vi "Send Parameter To ParameterDevice.vi"(8 "error in (no error)":errorcluster, 10 "Value":dbl, 11 "ExperimentService in":refnum<class "ExperimentService.lvclass">) -> (0 "error out":errorcluster, 3 "ExperimentService out":refnum<class "ExperimentService.lvclass">)   [LabVIEW 2014, in "ExperimentService.lvclass"]
uses:
  ExperimentService.lvclass
  ExperimentService Messages/Start ExperimentSet Msg/Start Experiment Set Msg.lvclass
  Hardware/ParameterDevice/ParameterDevice Messages/Set Parameter Msg/Set Parameter Msg.lvclass
  Model/Data/DataSingleElement/DataSingleElement.lvclass
  <vilib>/ActorFramework/Actor/Actor.lvclass/Actor.ctl
  <vilib>/ActorFramework/Message Enqueuer/Message Enqueuer.lvclass/Message Enqueuer.ctl
  ExperimentService.lvclass/ExperimentService.ctl
  Hardware/ParameterDevice/ParameterDevice Messages/Set Parameter Msg/Set Parameter Msg.lvclass/Set Parameter Msg.ctl
  <vilib>/ActorFramework/Message Enqueuer/Init from Existing Queue.vi
  <vilib>/ActorFramework/Message Enqueuer/Message Enqueuer.lvclass
  Replay Msg.lvclass
  <vilib>/ActorFramework/Actor/Actor.lvclass
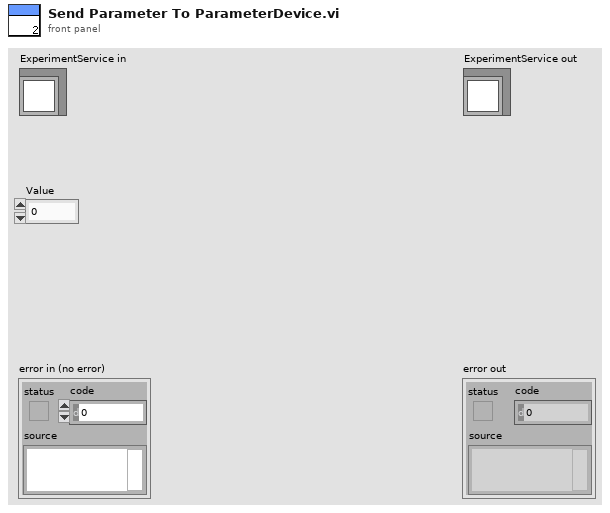
[diagram p1: front panel]
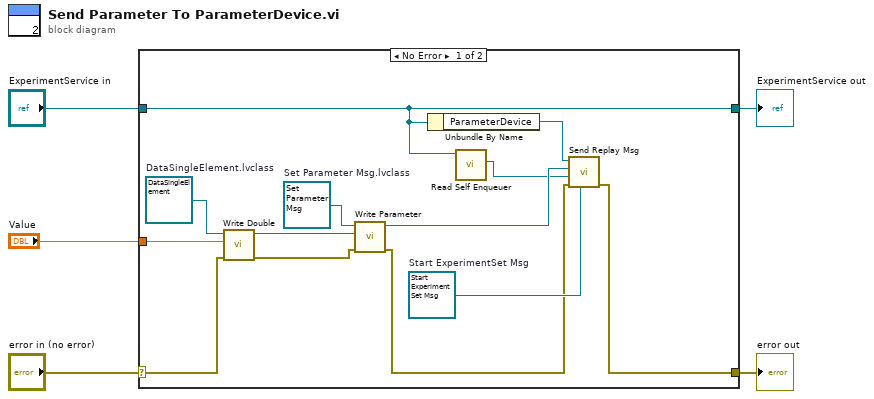
[diagram p0: block diagram]
diagram:
  n1 = case shown="No Error" "error in (no error)" {
    selector: "error in (no error)" -> [w7 w20]
    tunnel: [w18 w20] -> w4
    tunnel: [w14 w19] -> w2
    tunnel: "ExperimentService in" -> [w14 w19]
    tunnel: "Value" -> [w6 _]
    frame No Error {
      w10 = refnum<class "DataSingleElement.lvclass"> refnum  # DataSingleElement.lvclass
      w17 = refnum<class "Set Parameter Msg.lvclass"> refnum  # Set Parameter Msg.lvclass
      w12 = refnum<class "Start Experiment Set Msg.lvclass"> refnum  # Start ExperimentSet Msg
      n2 = call "Write Double.vi"("error in (no error)"=w7, "value"=w6, "DataSingleElement in"=w10) -> ("error out"=w8:errorcluster, "DataSingleElement out"=w9:refnum<class "DataSingleElement.lvclass">)  [unwired: 7 in]
      n3 = call "Write Parameter.vi"("error in (no error)"=w8, "Parameter"=w9, "Set Parameter Msg in"=w17) -> ("error out"=w11:errorcluster, "Set Parameter Msg out"=w16:refnum<class "Set Parameter Msg.lvclass">)  [unwired: 7 in]
      n4 = Unbundle By Name(w14) -> ("ParameterDevice"=w13:refnum<class "Message Enqueuer.lvclass">)
      n5 = call <vilib>:"Read Self Enqueuer.vi"("Actor"=w14) -> ("Self Enqueuer"=w15:refnum<class "Message Enqueuer.lvclass">)  [unwired: 10 in]
      n6 = call "Send Replay Msg.vi"("On End Message"=w12, "error in (no error)"=w11, "Caller Enqueuer"=w15, "Replay Message in"=w16, "Message Enqueuer"=w13) -> ("error out"=w18:errorcluster)  [unwired: 5 in, 1 out]
    }
    frame Error {
    }
  }
  "error out" <- w4
  "ExperimentService out" <- w2
